vi "Read IProjectItemFactory.vi"(11 "ProjectItem in":refnum<class "ProjectItem.lvclass">) -> (2 "IProjectItemFactory":refnum<class "IProjectItemFactory.lvclass">, 3 "ProjectItem out":refnum<class "ProjectItem.lvclass">)   [LabVIEW 2016, in "ProjectItem.lvclass"]
uses:
  ProjectItem.lvclass
  IProjectItemFactory/IProjectItemFactory.lvclass
  ProjectItem.lvclass/ProjectItem.ctl
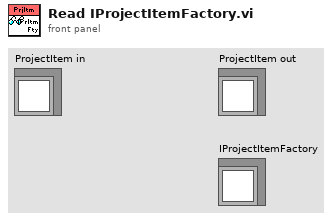
[diagram p1: front panel]
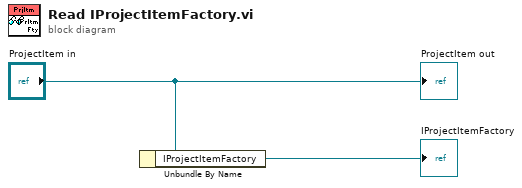
[diagram p0: block diagram]
diagram:
  n1 = Unbundle By Name("ProjectItem in") -> ("IProjectItemFactory"=→"IProjectItemFactory":refnum<class "IProjectItemFactory.lvclass">)
  "ProjectItem out" <- "ProjectItem in"
